vi "X cursor Read.vi"(4 "error in (no error)":errorcluster, 6 "Container State":T2, 7 "Display State In":T1={"X cursor"={"state"=enum."cursor and slider", "color"=6618880}, "Y cursor"={"state"=enum."cursor and slider", "color"=6618880}, "Scale Sliders"=FALSE}) -> (0 "error out":errorcluster, 2 "Value":T3={"state"=enum."cursor and slider", "color"=6618880}, 3 "Display State Out":T1={"X cursor"={"state"=enum."cursor and slider", "color"=6618880}, "Y cursor"={"state"=enum."cursor and slider", "color"=6618880}, "Scale Sliders"=FALSE})   [LabVIEW 2016, in "CursorImageControl.xctl"]
uses:
  CursorImageControl.xctl
  <vilib>/_xctls/Container State.ctl
  State.ctl
  <vilib>/_xctls/XControlSupport.lvlib
panel:
  # "Replace the Value Indicator below with an Indicator of desired type.\nDo not remove this Indicator or the others from the connector pane. \nDo not change the connector pane pattern.\nThe Value Indicator should always be the second terminal from top on the output side in the connector pane."
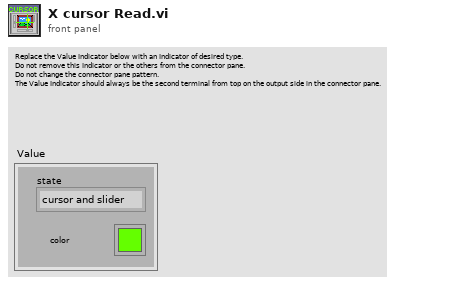
[diagram p1: front panel]
types:
  T1 = typedef "CursorImageControl.xctl/State.ctl" = cluster{"X cursor":cluster{"state":enum16{"cursor and slider", "cursor only", "hide all"}, "color":u32}, "Y cursor":cluster{"state":enum16{"cursor and slider", "cursor only", "hide all"}, "color":u32}, "Scale Sliders":bool}
  T2 = typedef "XControlSupport.lvlib/Container State.ctl" = cluster{"Indicator?":bool, "Run Mode?":bool, " Refnum":refnum<vi>}
  T3 = cluster{"state":enum16{"cursor and slider", "cursor only", "hide all"}, "color":u32}
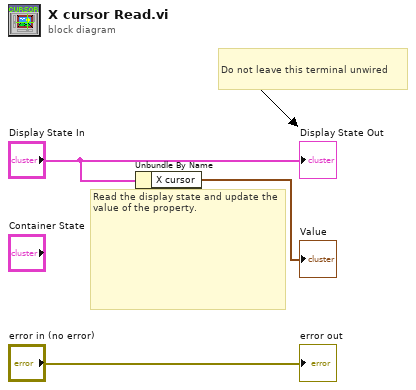
[diagram p0: block diagram]
diagram:
  # "Do not leave this terminal unwired"
  # "Read the display state and update the value of the property."
  n1 = Unbundle By Name("Display State In") -> ("X cursor"=→"Value":T3)
  "error out" <- "error in (no error)"
  "Display State Out" <- "Display State In"
